vi "Autotest.vi"(8 "error in (no error)":errorcluster caption="entrée d'erreur (pas d'erreur)", 11 "Power_Supply (Default) en entrée":refnum<class "Power_Supply (Default).lvclass">) -> (0 "error out":errorcluster caption="sortie d'erreur", 2 "Autotest Ok ?":bool, 3 "Power_Supply (Default) en sortie":refnum<class "Power_Supply (Default).lvclass">)   [LabVIEW 2020, in "Library Instrument & Equipement.lvlib" / "Library Power_Supply.lvlib" / "Power_Supply (Default).lvclass"]
uses:
  Power_Supply (Default).lvclass
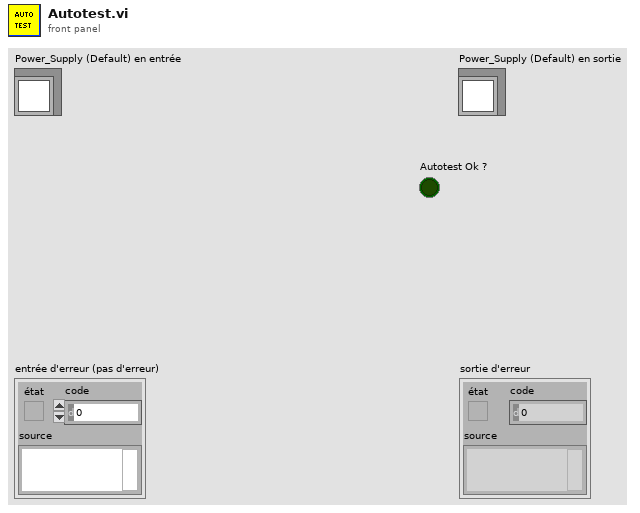
[diagram p1: front panel]
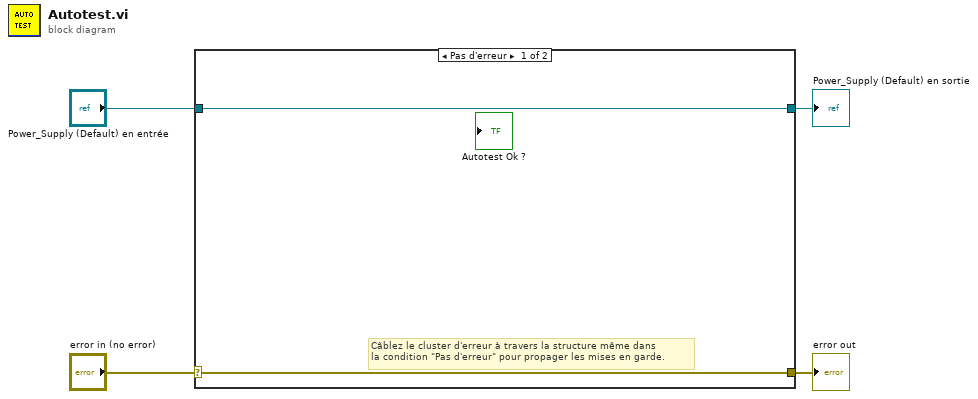
[diagram p0: block diagram]
diagram:
  n1 = case shown="Pas d'erreur" "error in (no error)" {
    selector: "error in (no error)" -> [w5 w8]
    tunnel: [w5 w8] -> w3
    tunnel: [w6 w7] -> w1
    tunnel: "Power_Supply (Default) en entrée" -> [w6 w7]
    frame No Error {
      # "Câblez le cluster d'erreur à travers la structure même dans\nla condition \"Pas d'erreur\" pour propager les mises en garde."
    }
    frame Error {
    }
  }
  "error out" <- w3
  "Power_Supply (Default) en sortie" <- w1
